vi "createSnapper.vi"(8 "error in (no error)":errorcluster, 9 "close":refnum<user-event>, 10 "snapperEvents":T1) -> (0 "error out":errorcluster, 3 "Snapper out":refnum<class "Snapper.lvclass">)   [LabVIEW 2009, in "Views.lvlib" / "Camera.lvlib" / "Snapper.lvclass"]
uses:
  Snapper.lvclass
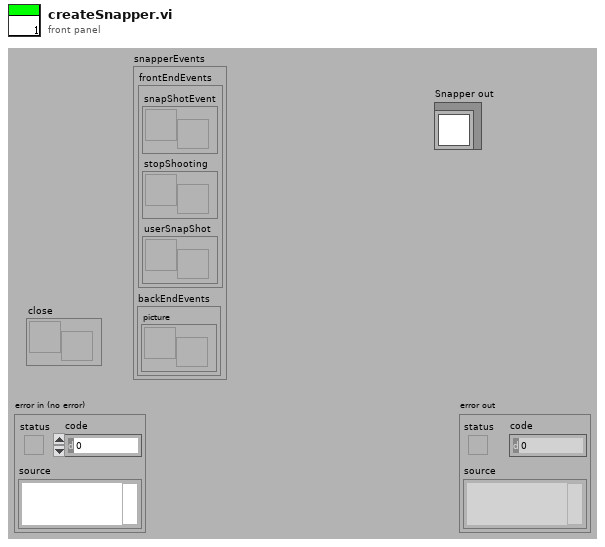
[diagram p1: front panel]
types:
  T1 = cluster{"frontEndEvents":cluster{"snapShotEvent":refnum<user-event>, "stopShooting":refnum<user-event>, "userSnapShot":refnum<user-event>}, "backEndEvents":cluster{"picture":refnum<user-event>}}
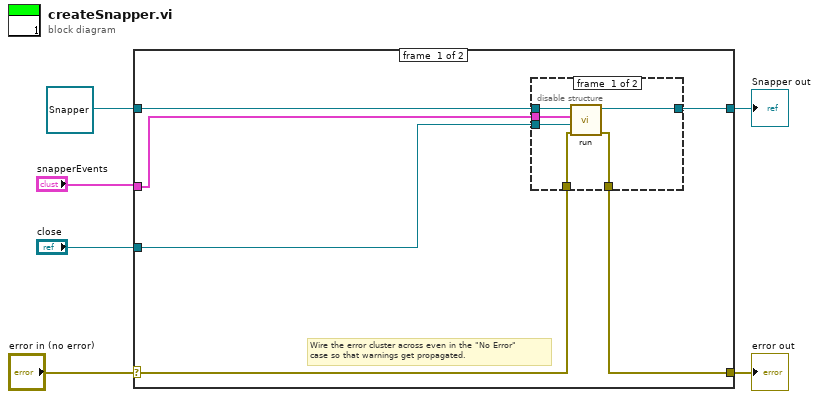
[diagram p0: block diagram]
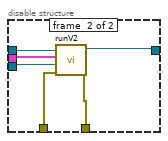
[diagram p2: hidden frame]
diagram:
  n1 = case shown="No Error" "error in (no error)" {
    selector: "error in (no error)" -> [w11 w26]
    tunnel: [w10 w26] -> w5
    tunnel: [w12 w25] -> w4
    tunnel: refnum<class "Snapper.lvclass"> refnum ("Views.lvlib:Camera.lvlib:Snapper.lvclass") -> [w9 w25]
    tunnel: "snapperEvents" -> [w7 _]
    tunnel: "close" -> [w8 _]
    frame #0 {
      # "Wire the error cluster across even in the \"No Error\"\ncase so that warnings get propagated."
      n2 = disable-structure shown="Enabled" {
        disable-tunnel: [w18 w23] -> w12
        disable-tunnel: w11 -> [w17 w22]
        disable-tunnel: [w16 w21] -> w10
        disable-tunnel: w9 -> [w15 w24]
        disable-tunnel: w8 -> [w14 w19]
        disable-tunnel: w7 -> [w13 w20]
        frame #0 {
          n3 = call-dynamic "run.vi"("error in (no error)"=w17, "closeEvent"=w14, "snapperEvents"=w13, "Views.lvlib:Camera.lvlib:Snapper in"=w15) -> ("error out"=w16:errorcluster, "Views.lvlib:Camera.lvlib:Snapper out"=w18:refnum<class "Snapper.lvclass">)  [unwired: 6 in]
        }
        frame #1 {
          n4 = call-dynamic "runV2.vi"("error in (no error)"=w22, "closeEvent"=w19, "snapperEvents"=w20, "Views.lvlib:Camera.lvlib:Snapper in"=w24) -> ("error out"=w21:errorcluster, "Views.lvlib:Camera.lvlib:Snapper out"=w23:refnum<class "Snapper.lvclass">)  [unwired: 6 in]
        }
      }
    }
    frame #1 {
    }
  }
  "error out" <- w5
  "Snapper out" <- w4
